vi "Automatic Teller Machine (ATM).vi"() -> ()   [LabVIEW 8.6]
doc: "This is a simulation of an Automated Teller Machine (ATM). It provides functionality for runtime-defined menus and functions, ATM card insertion and removal, and error handling."
uses:
  Controls/State.ctl
  Controls/Function.ctl
  Controls/Menu.ctl
  Controls/Buttons.ctl
panel:
  in  "Right Buttons":T1
  out "Right Menu":T2
  out "Left Menu":T2
  out "ATM Messages":string
  in  "User Input":string
  in  "Enter":bool
  in  "Left Buttons":T1
  in  "Card Simulator":bool
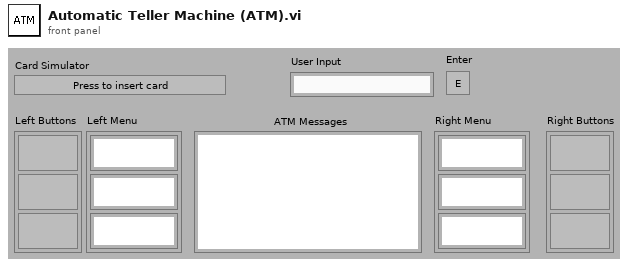
[diagram p1: front panel]
types:
  T1 = typedef "Buttons.ctl" = cluster{"Button 0":bool, "Button 1":bool, "Button 2":bool}
  T2 = typedef "Menu.ctl" = cluster{"Menu 0":string, "Menu 1":string, "Menu 2":string}
  T3 = typedef "State.ctl" = enum16{"Init", "Run", "Shutdown"}
  T4 = cluster{"User Input":refnum<vi>, "Left Buttons":refnum<vi>, "Right Buttons":refnum<vi>, "Enter":refnum<vi>, "Left Menu":refnum<vi>, "Right Menu":refnum<vi>, "Card Simulator":refnum<vi>, "ATM Messages":refnum<vi>}
  T5 = enum16{"Init", "Get Balance", "Update Balance", "Find Name"}
  T6 = enum8{"Enabled", "Disabled", "Disabled and Grayed Out"}
  T7 = typedef "Function.ctl" = string
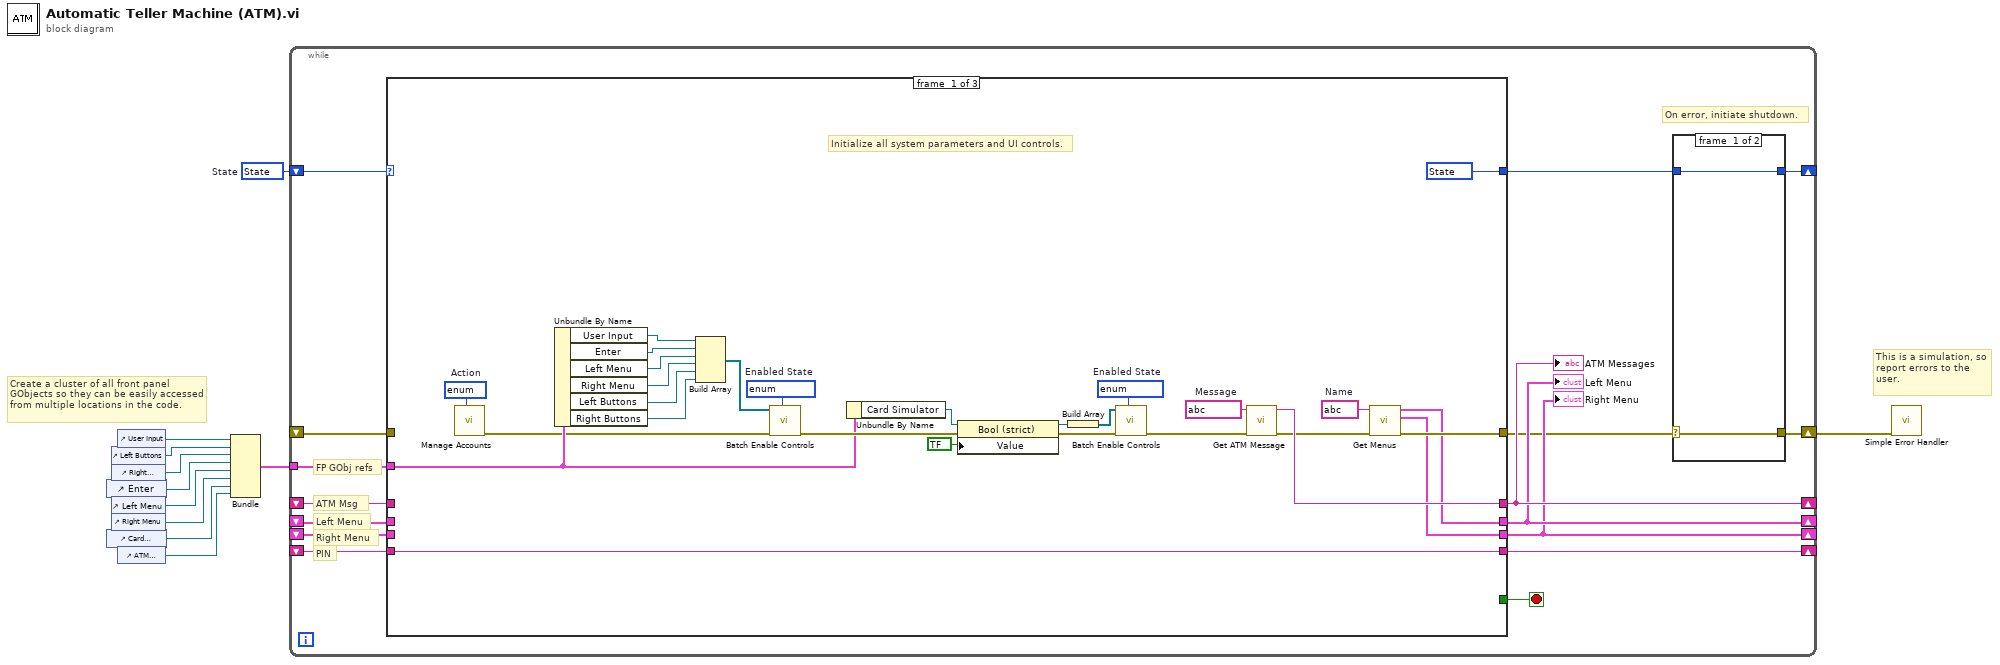
[diagram p0: block diagram]
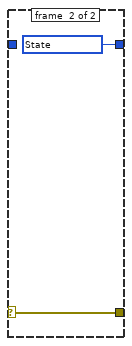
[diagram p2: hidden frame]
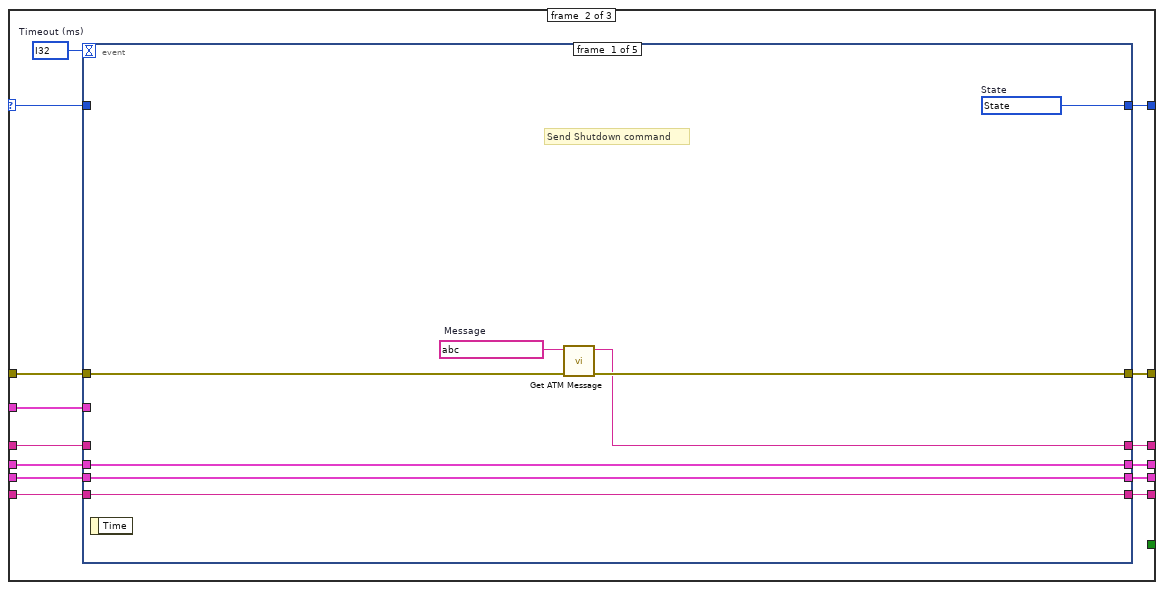
[diagram p3: hidden frame]
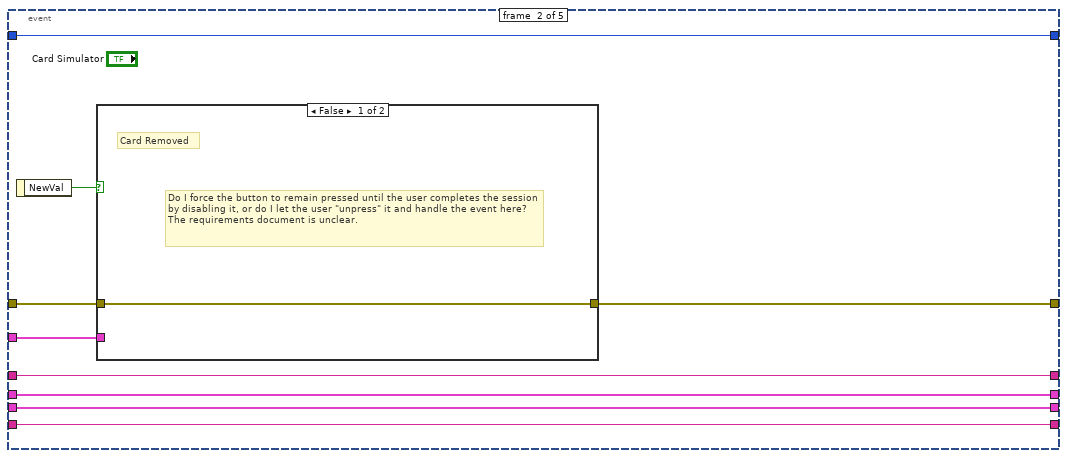
[diagram p4: hidden frame]
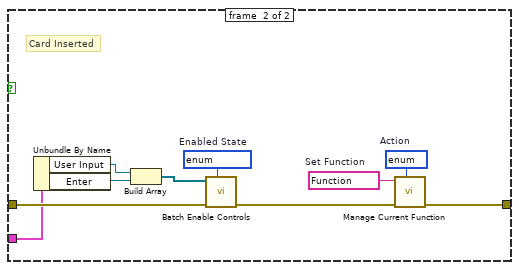
[diagram p5: hidden frame]
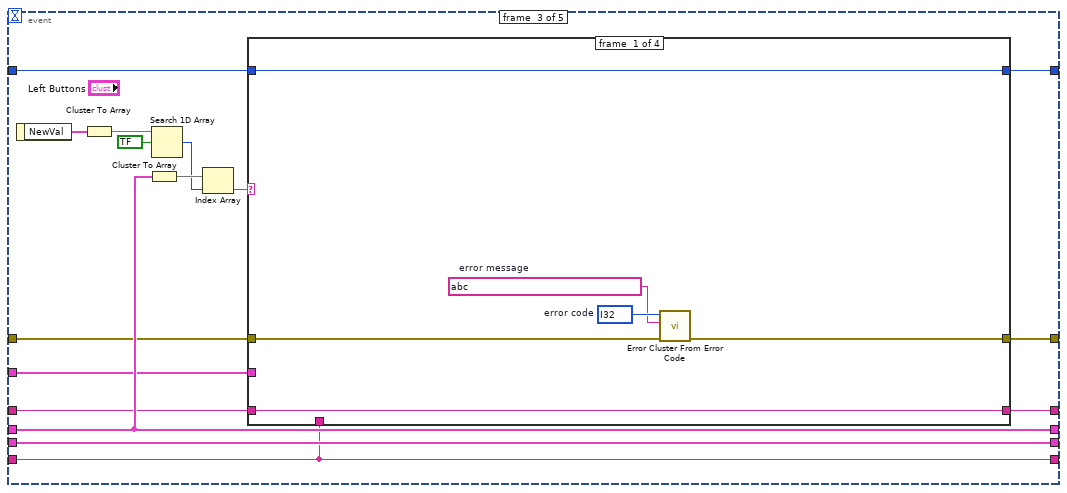
[diagram p6: hidden frame]
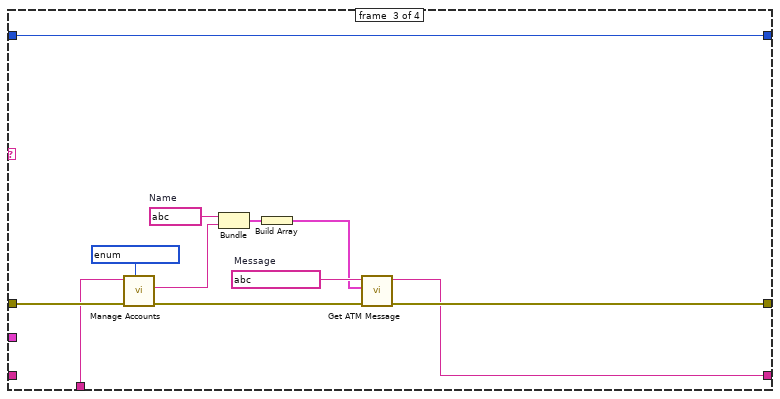
[diagram p8: hidden frame]
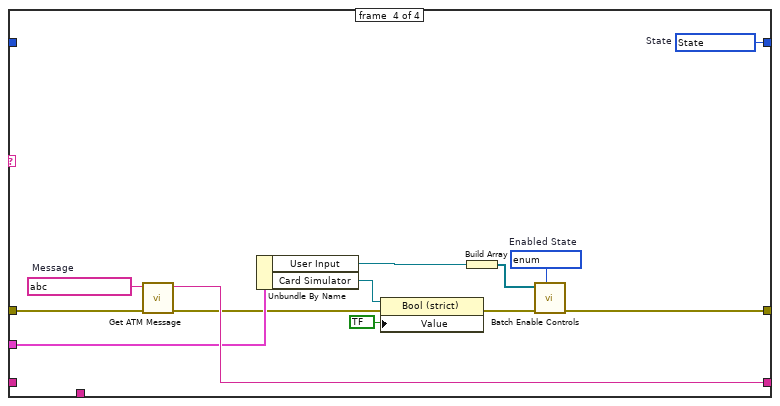
[diagram p9: hidden frame]
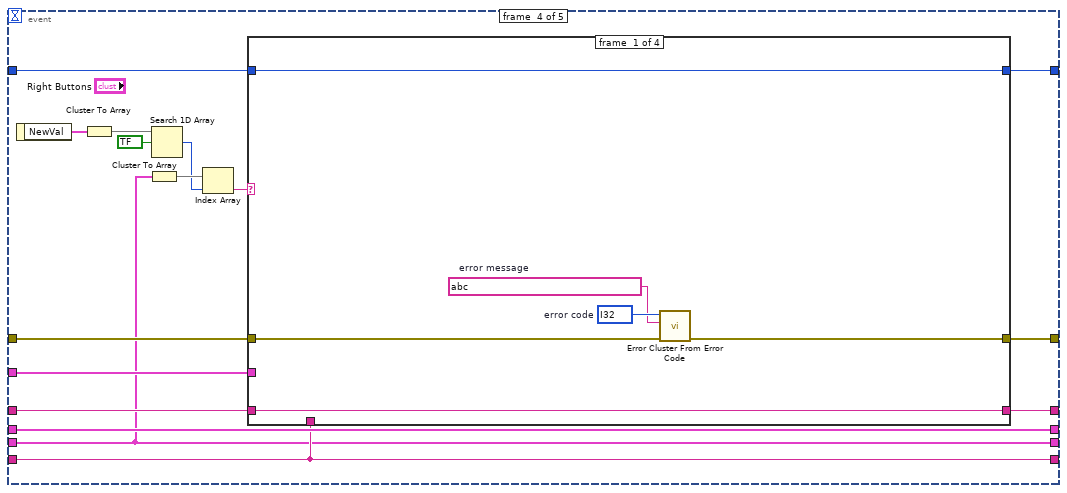
[diagram p10: hidden frame]
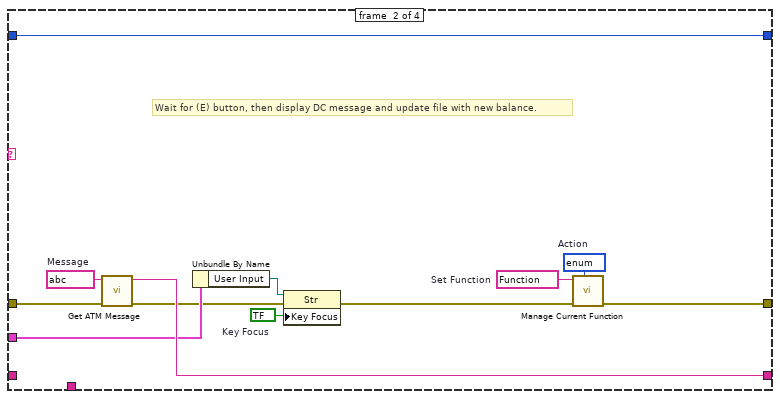
[diagram p11: hidden frame]
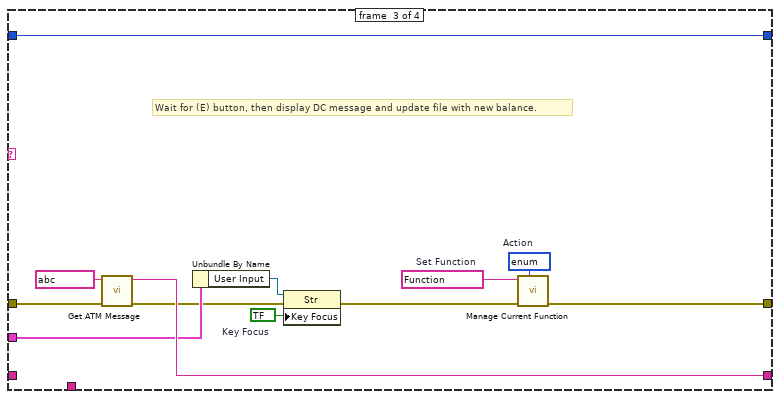
[diagram p12: hidden frame]
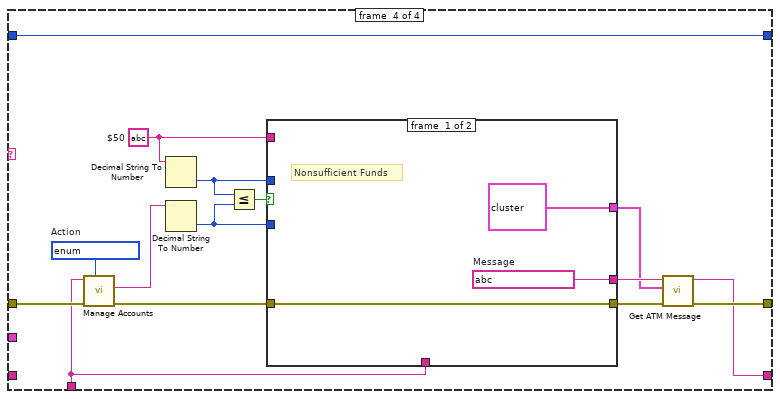
[diagram p13: hidden frame]
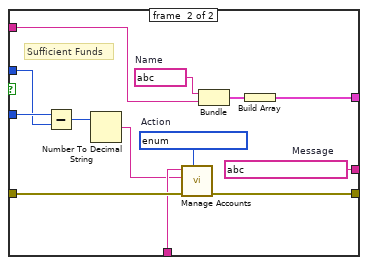
[diagram p14: hidden frame]
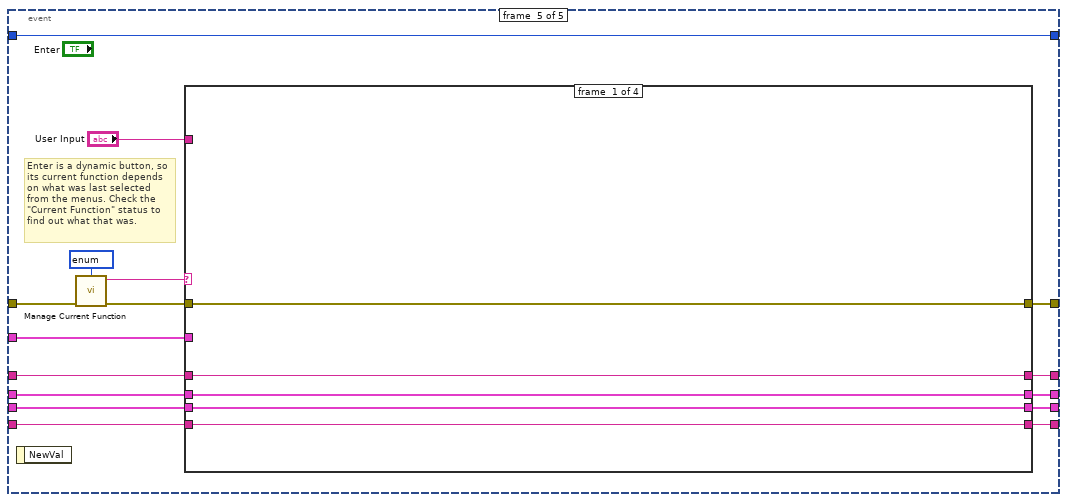
[diagram p15: hidden frame]
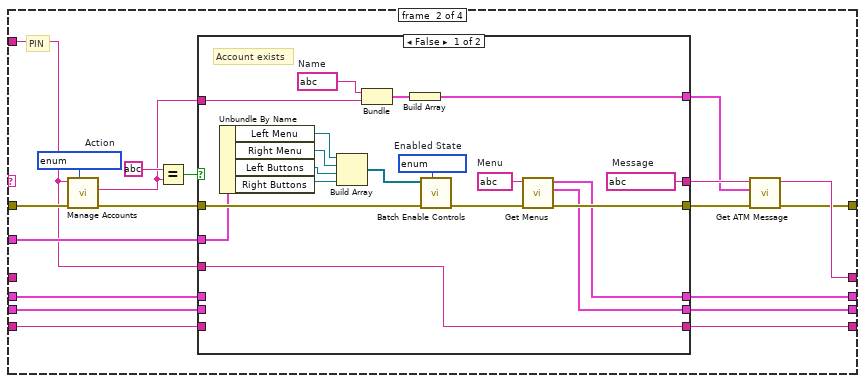
[diagram p16: hidden frame]
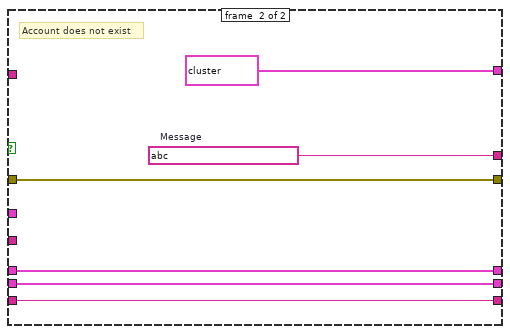
[diagram p17: hidden frame]
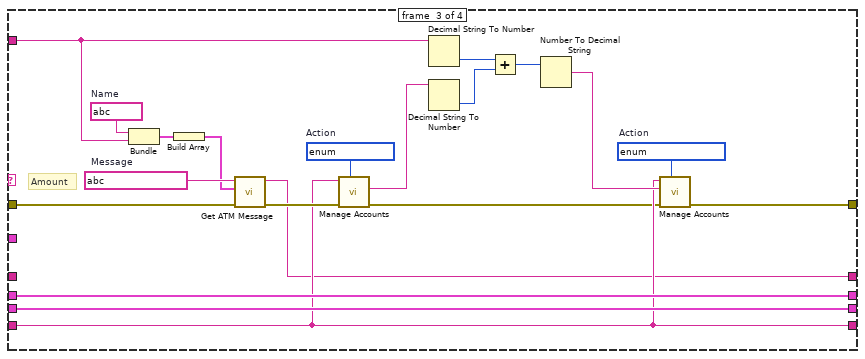
[diagram p18: hidden frame]
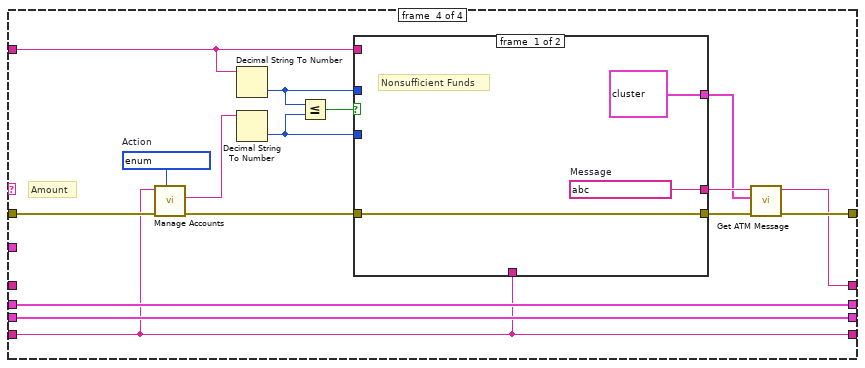
[diagram p19: hidden frame]
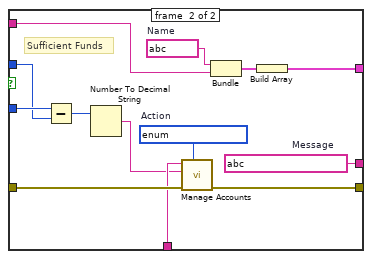
[diagram p20: hidden frame]
diagram:
  w11 = T3 ?  # State
  # "Create a cluster of all front panel GObjects so they can be easily accessed from multiple locations in the code."
  # "This is a simulation, so report errors to the user."
  n1 = control-ref of="Enter"() -> (w7:refnum<vi>)
  n2 = control-ref of="Card Simulator"() -> (w4:refnum<vi>)
  n3 = control-ref of="Left Buttons"() -> (w9:refnum<vi>)
  n4 = control-ref of="Right Buttons"() -> (w8:refnum<vi>)
  n5 = control-ref of="Left Menu"() -> (w6:refnum<vi>)
  n6 = control-ref of="Right Menu"() -> (w5:refnum<vi>)
  n7 = control-ref of="User Input"() -> (w10:refnum<vi>)
  n8 = control-ref of="ATM Messages"() -> (w3:refnum<vi>)
  n9 = Bundle("User Input"=w10, "Left Buttons"=w9, "Right Buttons"=w8, "Enter"=w7, "Left Menu"=w6, "Right Menu"=w5, "Card Simulator"=w4, "ATM Messages"=w3) -> (w2:T4)  [unwired: 1 in]
  n10 = while {
    shift-right: [w14] -> w1
    shift-left: _ -> [w27]
    shift-right: [w12] -> _
    shift-left: w11 -> [w26]
    tunnel: w2 -> [w25]
    shift-right: [w24] -> _
    shift-left: _ -> [w23]
    shift-right: [w20] -> _
    shift-left: _ -> [w22]
    shift-right: [w19] -> _
    shift-left: _ -> [w21]
    shift-right: [w18] -> _
    shift-left: _ -> [w17]
    stop <- w16 stop-if-true
    # "On error, initiate shutdown."
    # "PIN"
    # "Right Menu"
    # "Left Menu"
    # "ATM Msg"
    # "FP GObj refs"
    n11 = case shown="\"Run\"" w26 {
      selector: w26 -> [_ w60 w360]
      tunnel: [w39 w71 w346] -> w15
      tunnel: w27 -> [_ w72 w358]
      tunnel: [T3 ? ("State") w61 w360] -> w13
      tunnel: w25 -> [w45 w70 w357]
      tunnel: [w44 w68 w364] -> w24
      tunnel: w23 -> [_ w69 w364]
      tunnel: [w38 w67 w363] -> w19
      tunnel: [w37 w66 w362] -> w20
      tunnel: w22 -> [_ w65 w362]
      tunnel: w21 -> [_ w64 w363]
      tunnel: [w36 w63 w361] -> w18
      tunnel: w17 -> [w36 w62 w361]
      tunnel: [_ _ bool ?] -> w16
      frame #0 {
        w41 = string ?  # Name
        w42 = T5 ?  # Action
        w53 = T6 ?  # Enabled State
        w56 = T6 ?  # Enabled State
        w59 = string ?  # Message
        # "Initialize all system parameters and UI controls."
        n12 = call "Manage Accounts.vi"("Action"=w42) -> ("error out"=w43:errorcluster)  [unwired: 9 in, 1 out]
        n13 = Unbundle By Name(w45) -> ("User Input"=w51:refnum<vi>, "Enter"=w50:refnum<vi>, "Left Menu"=w49:refnum<vi>, "Right Menu"=w48:refnum<vi>, "Left Buttons"=w47:refnum<vi>, "Right Buttons"=w46:refnum<vi>)
        n14 = Build Array(w51, w50, w49, w48, w47, w46) -> (w58:refnum<vi>[])
        n15 = call "Batch Enable Controls.vi"("Enabled State"=w56, "error in (no error)"=w43, "GObject:Control Refnums"=w58) -> ("error out"=w55:errorcluster)  [unwired: 8 in]
        n16 = Unbundle By Name(w45) -> ("Card Simulator"=w34:refnum<vi>)
        n17 = property class="Bool (strict)"(reference=w34, error in=w55, "Value"=bool ?) -> (reference out=w33:refnum<vi>, error out=w35:errorcluster)
        n18 = Build Array(w33) -> (w54:refnum<vi>[])
        n19 = call "Batch Enable Controls.vi"("Enabled State"=w53, "error in (no error)"=w35, "GObject:Control Refnums"=w54) -> ("error out"=w52:errorcluster)  [unwired: 8 in]
        n20 = call "Get ATM Message.vi"("error in (no error)"=w52, "Message"=w59) -> ("error out"=w40:errorcluster, "String"=w44:string)  [unwired: 8 in]
        n21 = call "Get Menus.vi"("error in (no error)"=w40, "Name"=w41) -> ("error out"=w39:errorcluster, "Right Menu"=w38:T2, "Left Menu"=w37:T2)  [unwired: 7 in]
      }
      frame #1 {
        w73 = i32 ?  # Timeout (ms)
        n22 = event shown="[4] \"Enter\": Value Change" {
          selector: _ -> [_ _ _ _ _]
          dyn-events: _ -> [_ _ _ _ _]
          timeout: w73 -> [_ _ _ _ _]
          tunnel: w72 -> [w81 w89 w110 w160 w230]
          tunnel: [w80 w88 w109 w159 w241] -> w71
          tunnel: w70 -> [_ w87 w106 w156 w243]
          tunnel: w69 -> [_ w86 w107 w157 w232]
          tunnel: [w78 w86 w108 w158 w242] -> w68
          tunnel: [w75 w83 w105 w152 w240] -> w67
          tunnel: [w76 w84 w114 w164 w239] -> w66
          tunnel: w65 -> [w76 w84 w114 w164 w238]
          tunnel: w64 -> [w75 w83 w105 w152 w237]
          tunnel: [w77 w85 w104 w155 w234] -> w63
          tunnel: w62 -> [w77 w85 w104 w155 w233]
          tunnel: [w74 w82 w103 w154 w231] -> w61
          tunnel: w60 -> [_ w82 w102 w153 w231]
          event #0 {
            w74 = T3 ?  # State
            w79 = string ?  # Message
            # "Send Shutdown command"
            n23 = event-data() -> ()  [unwired: 1 in, 1 out]
            n24 = call "Get ATM Message.vi"("error in (no error)"=w81, "Message"=w79) -> ("error out"=w80:errorcluster, "String"=w78:string)  [unwired: 8 in]
          }
          event #1 {
            n25 = event-data() -> ("NewVal"=w90:bool)  [unwired: 1 in]
            n26 = case shown="False" w90 {
              tunnel: w89 -> [w91 w101]
              tunnel: [w91 w92] -> w88
              tunnel: w87 -> [_ w99]
              frame #0 {
                # "Do I force the button to remain pressed until the user completes the session by disabling it, or do I let the user \"unpress\" it and handle the event here? The requirements document is unclear."
                # "Card Removed"
              }
              frame #1 {
                w96 = T7 ?  # Set Function
                w97 = enum16{"Get", "Set"} ?  # Action
                w100 = T6 ?  # Enabled State
                # "Card Inserted"
                n27 = Unbundle By Name(w99) -> ("User Input"=w94:refnum<vi>, "Enter"=w95:refnum<vi>)
                n28 = Build Array(w94, w95) -> (w98:refnum<vi>[])
                n29 = call "Batch Enable Controls.vi"("Enabled State"=w100, "error in (no error)"=w101, "GObject:Control Refnums"=w98) -> ("error out"=w93:errorcluster)  [unwired: 8 in]
                n30 = call "Manage Current Function.vi"("Action"=w97, "error in (no error)"=w93, "Set Function"=w96) -> ("error out"=w92:errorcluster)  [unwired: 7 in, 1 out]
              }
            }
          }
          event #2 {
            n31 = event-data() -> ("NewVal"=w117:T1)  [unwired: 1 in]
            n32 = Cluster To Array(cluster=w117) -> (array=w116:bool[])
            n33 = Cluster To Array(cluster=w114) -> (array=w113:string[])
            n34 = Search 1D Array(1D array=w116, element=bool ?) -> (index of element=w112:i32)  [unwired: 1 in]
            n35 = Index Array(array=w113, index=w112) -> (element=w111:string)
            n36 = case shown="\"None\"" w111 {
              tunnel: w110 -> [w123 w126 w138 w151]
              tunnel: [w120 w126 w133 w139] -> w109
              tunnel: [w122 w125 w132 w149] -> w108
              tunnel: w107 -> [w122 w125 _ _]
              tunnel: w106 -> [_ _ _ w148]
              tunnel: w104 -> [_ _ w137 _]
              tunnel: [w121 w124 w127 w140] -> w103
              tunnel: w102 -> [w121 w124 w127 _]
              frame #0 {
                w118 = string ?  # error message
                w119 = i32 ?  # error code
                n37 = call <vilib>:"Error Cluster From Error Code.vi"("error in (no error)"=w123, "error message (\"\")"=w118, "error code (0)"=w119) -> ("error out"=w120:errorcluster)  [unwired: 6 in]
              }
              frame #1 {
                # "Reserved for future use. Do nothing."
              }
              frame #2 {
                w131 = string ?  # Name
                w134 = string ?  # Message
                n38 = call "Manage Accounts.vi"("Action"=T5 ?, "error in (no error)"=w138, "PIN"=w137) -> ("error out"=w135:errorcluster, "Get Value"=w130:string)  [unwired: 7 in]
                n39 = Bundle("Name"=w131, "Get Value"=w130) -> (w129:cluster{"Name":string, "Get Value":string})  [unwired: 1 in]
                n40 = Build Array(w129) -> (w128:cluster{"Name":string, "Get Value":string}[])
                n41 = call "Get ATM Message.vi"("error in (no error)"=w135, "Tokens"=w128, "Message"=w134) -> ("error out"=w133:errorcluster, "String"=w132:string)  [unwired: 7 in]
              }
              frame #3 {
                w140 = T3 ?  # State
                w143 = T6 ?  # Enabled State
                w150 = string ?  # Message
                n42 = call "Get ATM Message.vi"("error in (no error)"=w151, "Message"=w150) -> ("error out"=w147:errorcluster, "String"=w149:string)  [unwired: 8 in]
                n43 = Unbundle By Name(w148) -> ("User Input"=w142:refnum<vi>, "Card Simulator"=w146:refnum<vi>)
                n44 = property class="Bool (strict)"(reference=w146, error in=w147, "Value"=bool ?) -> (error out=w144:errorcluster)  [unwired: 1 out]
                n45 = Build Array(w142) -> (w141:refnum<vi>[])
                n46 = call "Batch Enable Controls.vi"("Enabled State"=w143, "error in (no error)"=w144, "GObject:Control Refnums"=w141) -> ("error out"=w139:errorcluster)  [unwired: 8 in]
              }
            }
          }
          event #3 {
            n47 = event-data() -> ("NewVal"=w167:T1)  [unwired: 1 in]
            n48 = Cluster To Array(cluster=w167) -> (array=w166:bool[])
            n49 = Cluster To Array(cluster=w152) -> (array=w163:string[])
            n50 = Search 1D Array(1D array=w166, element=bool ?) -> (index of element=w162:i32)  [unwired: 1 in]
            n51 = Index Array(array=w163, index=w162) -> (element=w161:string)
            n52 = case shown="\"Deposit\"" w161 {
              tunnel: w160 -> [w173 w185 w197 w204]
              tunnel: [w170 w174 w186 w203] -> w159
              tunnel: [w172 w183 w195 w202] -> w158
              tunnel: w157 -> [w172 _ _ _]
              tunnel: w156 -> [_ w182 w194 _]
              tunnel: w155 -> [_ _ _ w200]
              tunnel: [w171 w176 w188 w201] -> w154
              tunnel: w153 -> [w171 w176 w188 w201]
              frame #0 {
                w168 = string ?  # error message
                w169 = i32 ?  # error code
                n53 = call <vilib>:"Error Cluster From Error Code.vi"("error in (no error)"=w173, "error message (\"\")"=w168, "error code (0)"=w169) -> ("error out"=w170:errorcluster)  [unwired: 6 in]
              }
              frame #1 {
                w177 = T7 ?  # Set Function
                w178 = enum16{"Get", "Set"} ?  # Action
                w179 = bool ?  # Key Focus
                w184 = string ?  # Message
                # "Wait for (E) button, then display DC message and update file with new balance."
                n54 = call "Get ATM Message.vi"("error in (no error)"=w185, "Message"=w184) -> ("error out"=w180:errorcluster, "String"=w183:string)  [unwired: 8 in]
                n55 = Unbundle By Name(w182) -> ("User Input"=w181:refnum<vi>)
                n56 = property class="Str"(reference=w181, error in=w180, "Key Focus"=w179) -> (error out=w175:errorcluster)  [unwired: 1 out]
                n57 = call "Manage Current Function.vi"("Action"=w178, "error in (no error)"=w175, "Set Function"=w177) -> ("error out"=w174:errorcluster)  [unwired: 7 in, 1 out]
              }
              frame #2 {
                w189 = T7 ?  # Set Function
                w190 = enum16{"Get", "Set"} ?  # Action
                w191 = bool ?  # Key Focus
                # "Wait for (E) button, then display DC message and update file with new balance."
                n58 = call "Get ATM Message.vi"("error in (no error)"=w197, "Message"=string ?) -> ("error out"=w192:errorcluster, "String"=w195:string)  [unwired: 8 in]
                n59 = Unbundle By Name(w194) -> ("User Input"=w193:refnum<vi>)
                n60 = property class="Str"(reference=w193, error in=w192, "Key Focus"=w191) -> (error out=w187:errorcluster)  [unwired: 1 out]
                n61 = call "Manage Current Function.vi"("Action"=w190, "error in (no error)"=w187, "Set Function"=w189) -> ("error out"=w186:errorcluster)  [unwired: 7 in, 1 out]
              }
              frame #3 {
                w198 = string ?  # $50
                w212 = T5 ?  # Action
                n62 = call "Manage Accounts.vi"("Action"=w212, "error in (no error)"=w204, "PIN"=w200) -> ("error out"=w209:errorcluster, "Get Value"=w211:string)  [unwired: 7 in]
                n63 = Decimal String To Number(string=w198) -> (number=w208:i32)  [unwired: 2 in, 1 out]
                n64 = Decimal String To Number(string=w211) -> (number=w207:i32)  [unwired: 2 in, 1 out]
                n65 = Less Or Equal?(x=w208, y=w207) -> (x <= y?=w210:bool)
                n66 = case shown="True" w210 {
                  tunnel: w209 -> [w215 w225]
                  tunnel: [w215 w221] -> w206
                  tunnel: w208 -> [_ w227]
                  tunnel: w207 -> [_ w228]
                  tunnel: w200 -> [_ w224]
                  tunnel: [w214 w222] -> w205
                  tunnel: [cluster{string, string}[] ? w217] -> w199
                  tunnel: w198 -> [_ w216]
                  frame #0 {
                    w214 = string ?  # Message
                    # "Nonsufficient Funds"
                  }
                  frame #1 {
                    w219 = string ?  # Name
                    w222 = string ?  # Message
                    w226 = T5 ?  # Action
                    # "Sufficient Funds"
                    n67 = Subtract(x=w228, y=w227) -> (x-y=w223:i32)
                    n68 = Number To Decimal String(number=w223) -> (decimal integer string=w220:string)  [unwired: 1 in]
                    n69 = call "Manage Accounts.vi"("Action"=w226, "error in (no error)"=w225, "Set Value"=w220, "PIN"=w224) -> ("error out"=w221:errorcluster)  [unwired: 6 in, 1 out]
                    n70 = Bundle("Name"=w219, "$50"=w216) -> (w218:cluster{"Name":string, "$50":string})  [unwired: 1 in]
                    n71 = Build Array(w218) -> (w217:cluster{"Name":string, "$50":string}[])
                  }
                }
                n72 = call "Get ATM Message.vi"("error in (no error)"=w206, "Tokens"=w199, "Message"=w205) -> ("error out"=w203:errorcluster, "String"=w202:string)  [unwired: 7 in]
              }
            }
          }
          event #4 {
            # "Enter is a dynamic button, so its current function depends on what was last selected from the menus. Check the \"Current Function\" status to find out what that was."
            n73 = event-data() -> ()  [unwired: 1 in, 1 out]
            n74 = call "Manage Current Function.vi"("Action"=enum16{"Get", "Set"} ?, "error in (no error)"=w230) -> ("error out"=w229:errorcluster, "Get Function"=w235:T7)  [unwired: 8 in]
            n75 = case shown="\"Withdrawal\"" w235 {
              tunnel: w229 -> [w249 w268 w311 w326]
              tunnel: "User Input" -> [_ w252 w302 w315]
              tunnel: w243 -> [_ w264 _ _]
              tunnel: [w245 w262 w294 w317] -> w242
              tunnel: [w249 w257 w295 w318] -> w241
              tunnel: [w247 w256 w313 w329] -> w240
              tunnel: [w248 w255 w312 w328] -> w239
              tunnel: w238 -> [w248 w254 w312 w328]
              tunnel: w237 -> [w247 w253 w313 w329]
              tunnel: [w246 w251 w297 w320] -> w234
              tunnel: w233 -> [w246 w250 w297 w320]
              tunnel: w232 -> [w245 _ _ _]
              frame #0 {
              }
              frame #1 {
                w267 = T5 ?  # Action
                # "PIN"
                n76 = call "Manage Accounts.vi"("Action"=w267, "error in (no error)"=w268, "PIN"=w252) -> ("error out"=w266:errorcluster, "Get Value"=w258:string)  [unwired: 7 in]
                n77 = Equal?(x=string ?, y=w258) -> (x = y?=w265:bool)
                n78 = case shown="False" w265 {
                  tunnel: w266 -> [w287 w293]
                  tunnel: [w272 w293] -> w263
                  tunnel: w264 -> [w285 _]
                  tunnel: [w275 w292] -> w261
                  tunnel: [w276 cluster{"Name":string, "Value":string}[] ? ("Tokens")] -> w260
                  tunnel: w258 -> [w278 _]
                  tunnel: [w271 w289] -> w256
                  tunnel: [w270 w290] -> w255
                  tunnel: w254 -> [_ w290]
                  tunnel: w253 -> [_ w289]
                  tunnel: w252 -> [w269 _]
                  tunnel: [w269 w288] -> w251
                  tunnel: w250 -> [_ w288]
                  frame #0 {
                    w273 = string ?  # Menu
                    w279 = string ?  # Name
                    w275 = string ?  # Message
                    w286 = T6 ?  # Enabled State
                    # "Account exists"
                    n79 = Unbundle By Name(w285) -> ("Left Menu"=w280:refnum<vi>, "Right Menu"=w281:refnum<vi>, "Left Buttons"=w282:refnum<vi>, "Right Buttons"=w284:refnum<vi>)
                    n80 = Build Array(w280, w281, w282, w284) -> (w283:refnum<vi>[])
                    n81 = Bundle("Name"=w279, "Get Value"=w278) -> (w277:cluster{"Name":string, "Get Value":string})  [unwired: 1 in]
                    n82 = Build Array(w277) -> (w276:cluster{"Name":string, "Get Value":string}[])
                    n83 = call "Batch Enable Controls.vi"("Enabled State"=w286, "error in (no error)"=w287, "GObject:Control Refnums"=w283) -> ("error out"=w274:errorcluster)  [unwired: 8 in]
                    n84 = call "Get Menus.vi"("error in (no error)"=w274, "Name"=w273) -> ("error out"=w272:errorcluster, "Right Menu"=w271:T2, "Left Menu"=w270:T2)  [unwired: 7 in]
                  }
                  frame #1 {
                    w292 = string ?  # Message
                    # "Account does not exist"
                  }
                }
                n85 = call "Get ATM Message.vi"("error in (no error)"=w263, "Tokens"=w260, "Message"=w261) -> ("error out"=w257:errorcluster, "String"=w262:string)  [unwired: 7 in]
              }
              frame #2 {
                w305 = T5 ?  # Action
                w306 = T5 ?  # Action
                w309 = string ?  # Name
                w310 = string ?  # Message
                # "Amount"
                n86 = Bundle("Name"=w309, "User Input"=w302) -> (w308:cluster{"Name":string, "User Input":string})  [unwired: 1 in]
                n87 = Build Array(w308) -> (w307:cluster{"Name":string, "User Input":string}[])
                n88 = call "Get ATM Message.vi"("error in (no error)"=w311, "Tokens"=w307, "Message"=w310) -> ("error out"=w304:errorcluster, "String"=w294:string)  [unwired: 7 in]
                n89 = call "Manage Accounts.vi"("Action"=w305, "error in (no error)"=w304, "PIN"=w297) -> ("error out"=w296:errorcluster, "Get Value"=w303:string)  [unwired: 7 in]
                n90 = Decimal String To Number(string=w302) -> (number=w301:i32)  [unwired: 2 in, 1 out]
                n91 = Decimal String To Number(string=w303) -> (number=w300:i32)  [unwired: 2 in, 1 out]
                n92 = Add(x=w301, y=w300) -> (x+y=w299:i32)
                n93 = Number To Decimal String(number=w299) -> (decimal integer string=w298:string)  [unwired: 1 in]
                n94 = call "Manage Accounts.vi"("Action"=w306, "error in (no error)"=w296, "Set Value"=w298, "PIN"=w297) -> ("error out"=w295:errorcluster)  [unwired: 6 in, 1 out]
              }
              frame #3 {
                w327 = T5 ?  # Action
                # "Amount"
                n95 = call "Manage Accounts.vi"("Action"=w327, "error in (no error)"=w326, "PIN"=w320) -> ("error out"=w323:errorcluster, "Get Value"=w325:string)  [unwired: 7 in]
                n96 = Decimal String To Number(string=w315) -> (number=w322:i32)  [unwired: 2 in, 1 out]
                n97 = Decimal String To Number(string=w325) -> (number=w321:i32)  [unwired: 2 in, 1 out]
                n98 = Less Or Equal?(x=w322, y=w321) -> (x <= y?=w324:bool)
                n99 = case shown="True" w324 {
                  tunnel: w323 -> [w332 w342]
                  tunnel: [w332 w337] -> w319
                  tunnel: w322 -> [_ w344]
                  tunnel: w321 -> [_ w345]
                  tunnel: w320 -> [_ w341]
                  tunnel: [w331 w338] -> w316
                  tunnel: w315 -> [_ w334]
                  tunnel: [cluster{string, "User Input":string}[] ? w333] -> w314
                  frame #0 {
                    w331 = string ?  # Message
                    # "Nonsufficient Funds"
                  }
                  frame #1 {
                    w336 = string ?  # Name
                    w338 = string ?  # Message
                    w343 = T5 ?  # Action
                    # "Sufficient Funds"
                    n100 = Subtract(x=w345, y=w344) -> (x-y=w340:i32)
                    n101 = Number To Decimal String(number=w340) -> (decimal integer string=w339:string)  [unwired: 1 in]
                    n102 = call "Manage Accounts.vi"("Action"=w343, "error in (no error)"=w342, "Set Value"=w339, "PIN"=w341) -> ("error out"=w337:errorcluster)  [unwired: 6 in, 1 out]
                    n103 = Bundle("Name"=w336, "User Input"=w334) -> (w335:cluster{"Name":string, "User Input":string})  [unwired: 1 in]
                    n104 = Build Array(w335) -> (w333:cluster{"Name":string, "User Input":string}[])
                  }
                }
                n105 = call "Get ATM Message.vi"("error in (no error)"=w319, "Tokens"=w314, "Message"=w316) -> ("error out"=w318:errorcluster, "String"=w317:string)  [unwired: 7 in]
              }
            }
          }
        }
      }
      frame #2 {
        w347 = T6 ?  # Enabled State
        # "Return all controls to enabled state"
        n106 = Unbundle(w357) -> ("User Input"=w356:refnum<vi>, "Left Buttons"=w355:refnum<vi>, "Right Buttons"=w354:refnum<vi>, "Enter"=w353:refnum<vi>, "Left Menu"=w352:refnum<vi>, "Right Menu"=w351:refnum<vi>, "Card Simulator"=w350:refnum<vi>, "ATM Messages"=w349:refnum<vi>)
        n107 = Build Array(w356, w355, w354, w353, w352, w351, w350, w349) -> (w348:refnum<vi>[])
        n108 = call "Batch Enable Controls.vi"("Enabled State"=w347, "error in (no error)"=w358, "GObject:Control Refnums"=w348) -> ("error out"=w346:errorcluster)  [unwired: 8 in]
      }
    }
    "ATM Messages" <- w24
    "Left Menu" <- w20
    "Right Menu" <- w19
    n109 = case shown="Error" w15 {
      selector: w15 -> [w29 w30]
      tunnel: [w29 w30] -> w14
      tunnel: w13 -> [w28 _]
      tunnel: [w28 T3 ? ("State")] -> w12
      frame #0 {
      }
      frame #1 {
      }
    }
  }
  n110 = call <vilib>:"Simple Error Handler.vi"("error in (no error)"=w1) -> ()  [unwired: 4 in, 5 out]
